vi "DriveForTime-C.vi"(11 "Params":string[][](array[string])) -> ()   [LabVIEW 2020]
uses:
  Framework/Robot Global Data.vi
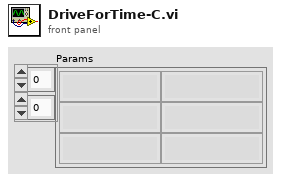
[diagram p1: front panel]
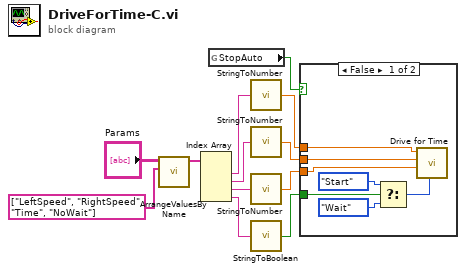
[diagram p0: block diagram]
diagram:
  n1 = call "ArrangeValuesByName.vi"("Names"=string[] ["LeftSpeed", "RightSpeed", "Time", "NoWait"], "Names/Values in"="Params") -> ("Values Out"=w5:string[])  [unwired: 9 in]
  n2 = Index Array(array=w5) -> (element #1=w4:string, element #2=w3:string, element #3=w2:string, element #4=w1:string)  [unwired: 4 in]
  n3 = global read "Robot Global Data.vi" "StopAuto"() -> (w12:bool)
  n4 = call "StringToNumber.vi"("String"=w4) -> ("Output"=w8:dbl)
  n5 = call "StringToNumber.vi"("String"=w3) -> ("Output"=w9:dbl)
  n6 = call "StringToNumber.vi"("String"=w2) -> ("Output"=w10:dbl)
  n7 = call "StringToBoolean.vi"("String"=w1) -> ("Output"=w11:bool)
  n8 = case shown="False" w12 {
    tunnel: w11 -> [w18 _]
    tunnel: w10 -> [w15 _]
    tunnel: w9 -> [w14 _]
    tunnel: w8 -> [w13 _]
    frame False {
      n9 = Select(t=enum16{"Start", "Wait"}."Start" ("Synchronization"), s=w18, f=enum16{"Start", "Wait"}."Wait" ("Synchronization")) -> (s? t:f=w16:enum16{"Start", "Wait"})
      n10 = call "Drive for Time.vi"("Synchronization"=w16, "Seconds"=w15, "Right Speed"=w14, "Left Speed"=w13) -> ()  [unwired: 7 in, 1 out]
    }
    frame True {
    }
  }
